vi "ObserverExample.vi"() -> ()   [LabVIEW 2025]
uses:
  ELT/Framework2.5/variantlib_code/Abstract_Actor/Abstract_Actor/Abstract_Actor.lvclass
  ELT/Framework2.5/variantlib_code/Abstract_Actor/Abstract_Actor/Abstract_Actor.lvclass/Abstract_Actor.ctl
  1c3370e3-be76-47c4-a4df-425e48d24b20.vi
  <vilib>/Utility/Data Type/NI_Data Type.lvlib
  ELT/Framework2.5/variantlib/General_Support.lvlibp
panel:
  in  "ObserverEnable":bool
  out "actorDataChanged":bool
  out "observedDataChanged":bool[](array[boolean])
  out "Cluster_out":variant[](array[variant])
  out "allActorDataName":string[](array[string])
  in  "Sender":string="pippo"
  out "Loop2":T1(array[cluster])
  out "Loop1":T1(array[cluster])
  in  "stop":bool
  out "LiveDataNames":string[](array[string])
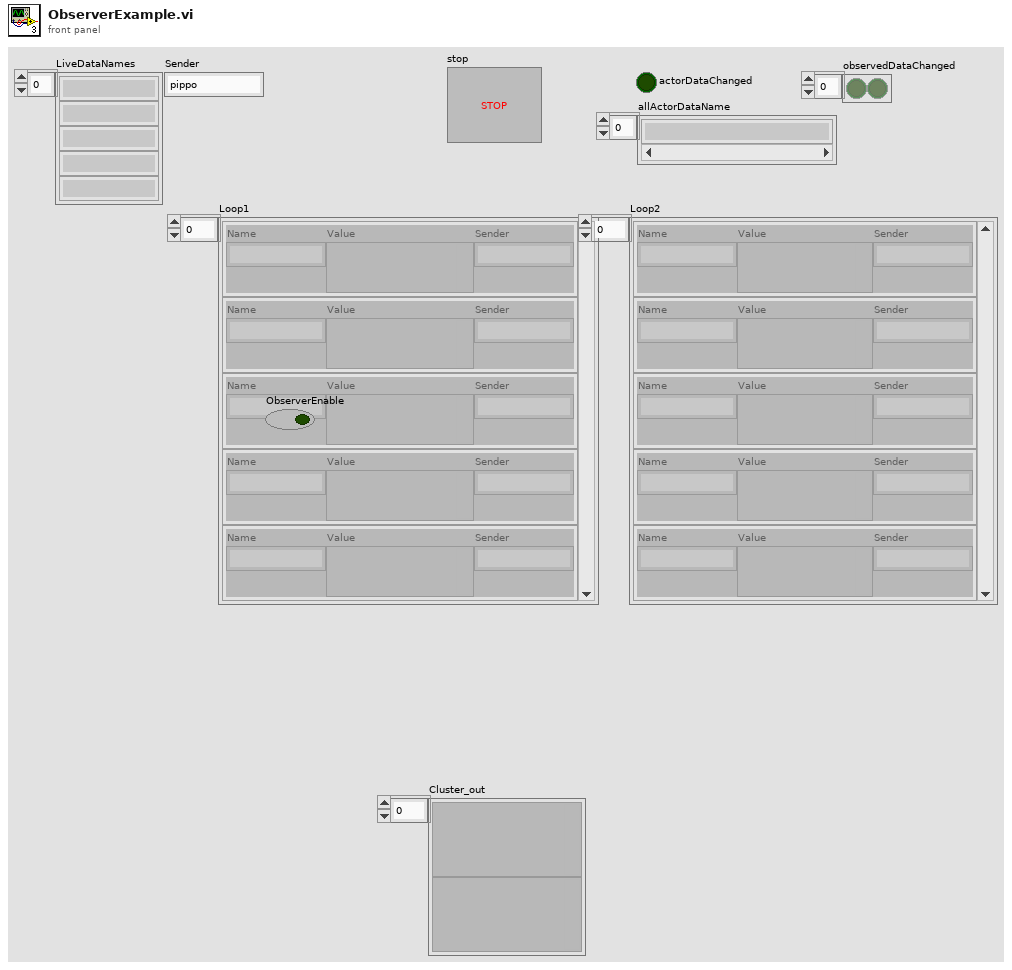
[diagram p1: front panel]
types:
  T1 = cluster{"Name":string, "Value":variant, "Sender":string}[]
  T2 = cluster{"Caller_Alias":string, "Actor_Alias":string}
  T3 = cluster{"Name":string, "Value":variant, "Sender":string}
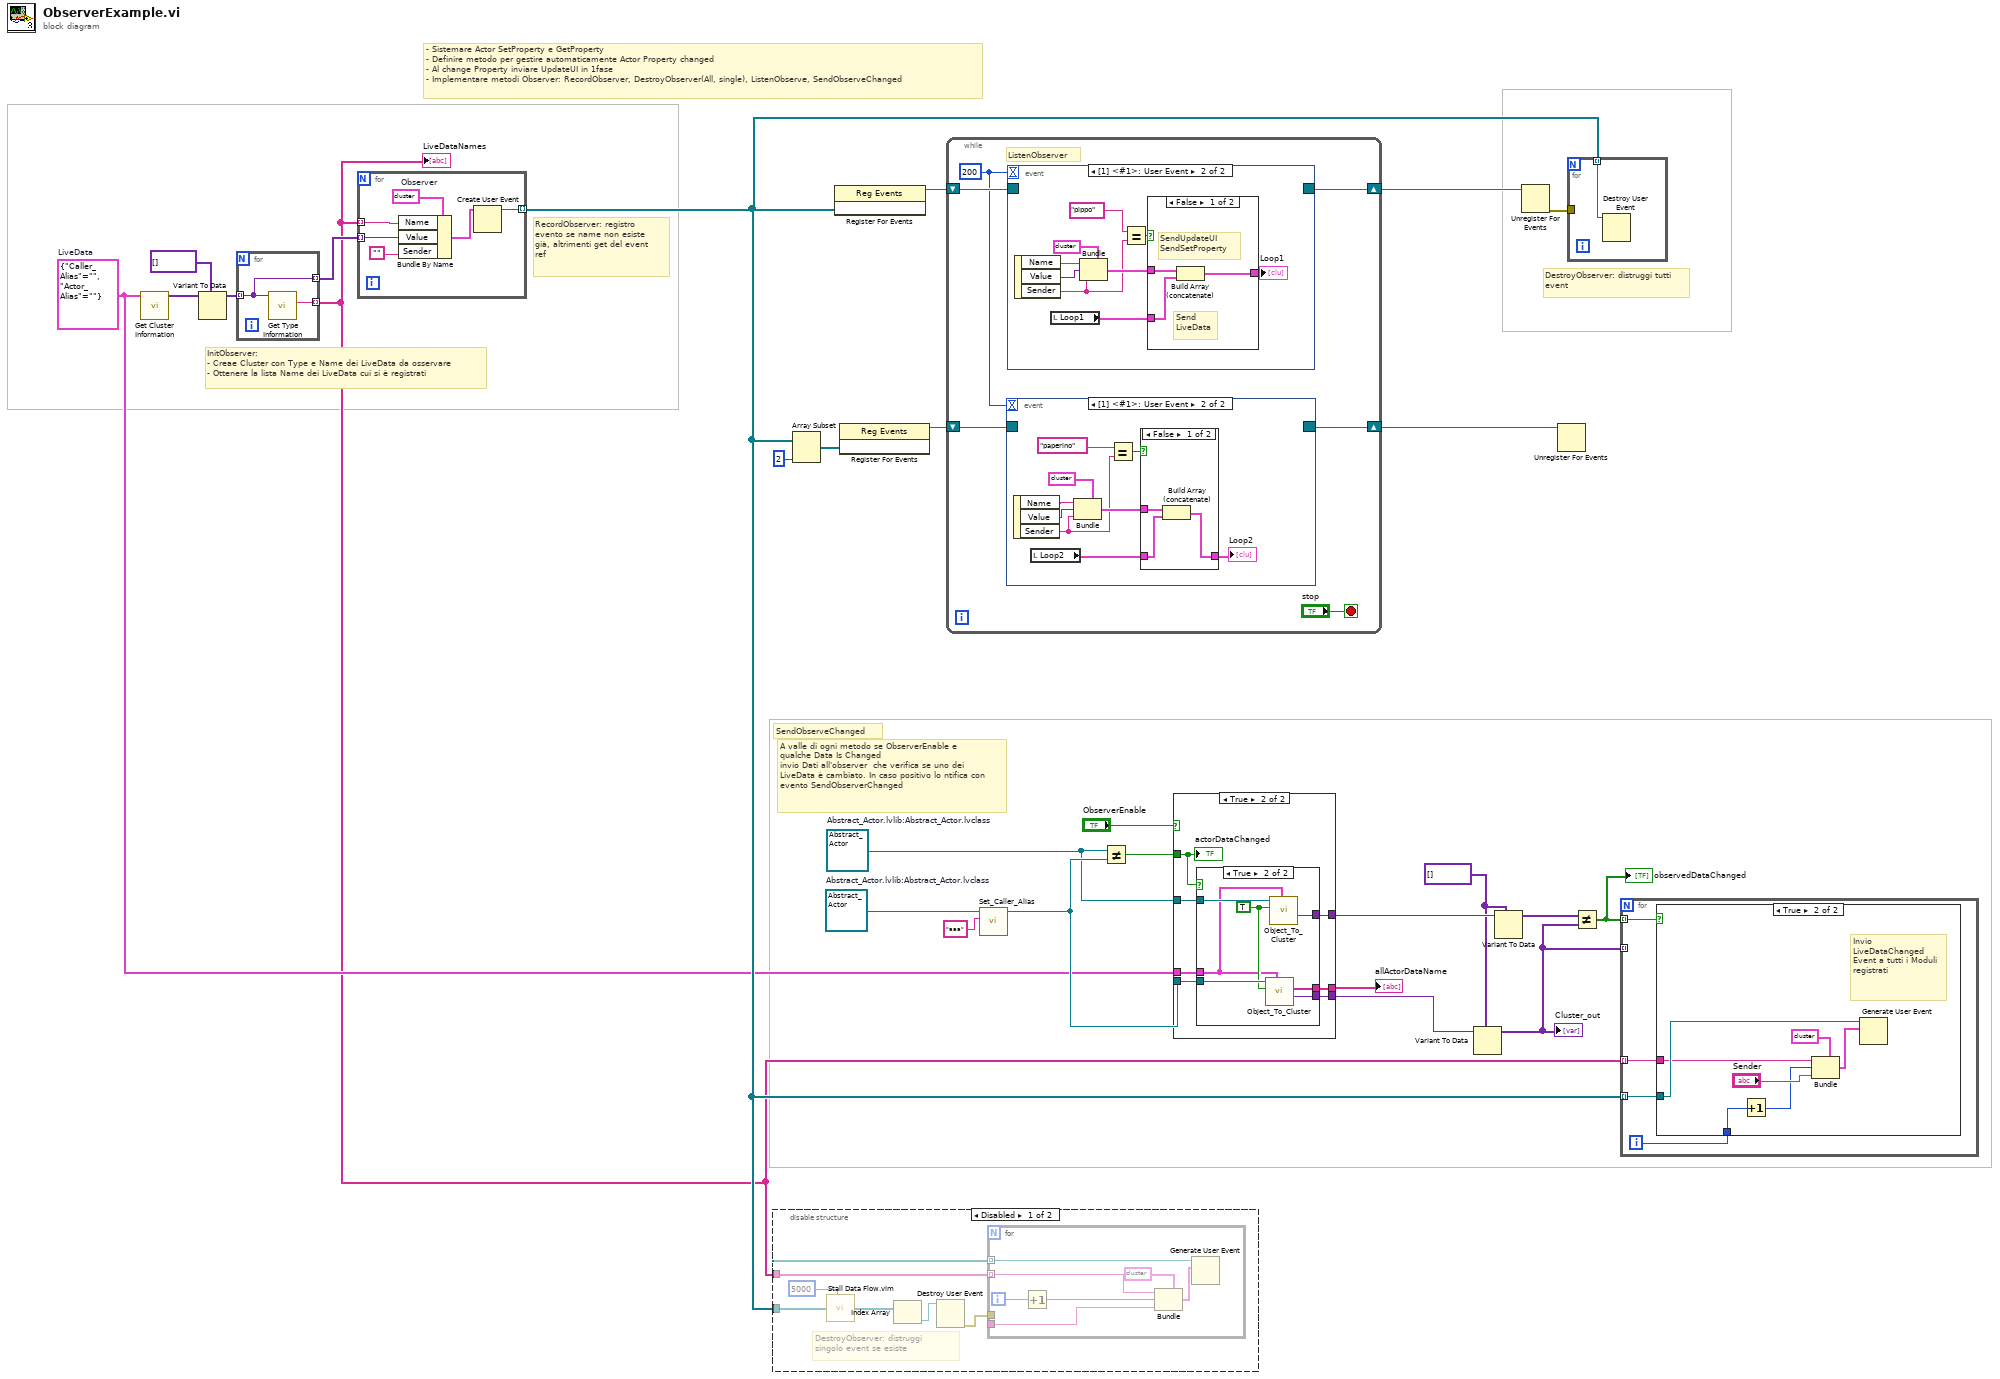
[diagram p0: block diagram]
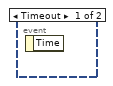
[diagram p5: hidden frame]
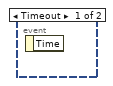
[diagram p7: hidden frame]
diagram:
  w8 = variant[] [] ("type")
  w15 = refnum<class "Abstract_Actor.lvclass"> refnum  # Abstract_Actor.lvlib:Abstract_Actor.lvclass
  w7 = refnum<class "Abstract_Actor.lvclass"> refnum  # Abstract_Actor.lvlib:Abstract_Actor.lvclass
  w2 = T2 {"Caller_Alias"="", "Actor_Alias"=""}  # LiveData
  # "A valle di ogni metodo se ObserverEnable e qualche Data Is Changed\ninvio Dati all'observer  che verifica se uno dei LiveData è cambiato. In caso positivo lo ntifica con evento SendObserverChanged"
  # "InitObserver:\n- Creae Cluster con Type e Name dei LiveData da osservare\n- Ottenere la lista Name dei LiveData cui si è registrati"
  # "SendObserveChanged"
  # "- Sistemare Actor SetProperty e GetProperty\n- Definire metodo per gestire automaticamente Actor Property changed\n- Al change Property inviare UpdateUI in 1fase\n- Implementare metodi Observer: RecordObserver, DestroyObserver(All, single), ListenObserve, SendObserveChanged"
  # "DestroyObserver: distruggi tutti event"
  # "RecordObserver: registro evento se name non esiste già, altrimenti get del event ref"
  n1 = call <vilib>:"Get Cluster Information.vi"("variant"=w2) -> ("cluster elements"=w20:variant[])  [unwired: 9 in, 1 out]
  n2 = Variant To Data(type=variant[] [], Variant=w20) -> (data=w18:variant[])  [unwired: 1 in, 1 out]
  n3 = for {
    tunnel: w18 -> [w28] mode=indexing
    tunnel: [w29] -> w1 mode=indexing
    tunnel: [w28] -> w17 mode=indexing
    n4 = call <vilib>:"Get Type Information.vi"("variant"=w28) -> ("name"=w29:string)  [unwired: 6 in, 4 out]
  }
  "LiveDataNames" <- w1
  n5 = for {
    tunnel: [w35] -> w3 mode=indexing
    tunnel: w1 -> [w33] mode=indexing
    tunnel: w17 -> [w31] mode=indexing
    w34 = T3 {"Name"="", "Value"=variant, "Sender"=""}  # Observer
    n6 = Bundle By Name(cluster=w34, "Name"=w33, "Value"=w31, "Sender"="") -> (w32:T3)
    n7 = Create User Event(user event datatype=w32) -> (user event=w35:refnum<user-event>)  [unwired: 1 in, 1 out]
  }
  n8 = disable-structure shown="Disabled" {
    disable-tunnel: w3 -> [w37 _]
    disable-tunnel: w1 -> [w36 _]
    frame Disabled {
      # "DestroyObserver: distruggi singolo event se esiste"
      n9 = call "Stall Data Flow.vim"("value in"=w37, "milliseconds to wait"=u32 5000) -> ("value out"=w40:refnum<user-event>[])  [unwired: 1 out]
      n10 = Index Array(array=w40) -> (element=w41:refnum<user-event>)  [unwired: 1 in]
      n11 = Destroy User Event(user event=w41) -> (error out=w38:errorcluster)  [unwired: 1 in]
      n12 = for {
        tunnel: w37 -> [w48] mode=indexing
        tunnel: w36 -> [w46] mode=indexing
        tunnel: w38 -> [_]
        tunnel: _ -> [w43]
        i -> [w47]
        n13 = Increment(x=w47) -> (x+1=w44:i32)
        n14 = Bundle(cluster=T3 {"Name"="", "Value"=variant, "Sender"=""} ("Observer"), "Name"=w46, "Value"=w44, "Sender"=w43) -> (w45:T3)
        n15 = Generate User Event(user event=w48, event data cluster=w45) -> ()  [unwired: 2 in, 2 out]
      }
    }
    frame Enabled {
    }
  }
  n16 = Array Subset(array=w3, length=2) -> (w22:refnum<user-event>[])  [unwired: 1 in]
  n17 = register-events(w3) -> (reference out=w25:refnum<event-registration>)  [unwired: 2 in, 1 out]
  n18 = register-events(w22) -> (reference out=w23:refnum<event-registration>)  [unwired: 2 in, 1 out]
  n19 = while {
    shift-right: [w54] -> w27
    shift-left: w25 -> [w53]
    shift-right: [w52] -> w24
    shift-left: w23 -> [w49]
    stop <- "stop" stop-if-true
    w50 = 200
    # "ListenObserver"
    n20 = event shown="[1] <#1>: User Event" {
      selector: w49 -> [_ _]
      dyn-events: [_ _] -> w52
      timeout: w50 -> [_ _]
      event Timeout {
        n21 = event-data() -> ()  [unwired: 1 in, 1 out]
      }
      event User Event {
        n22 = event-data() -> ("Name"=w62:string, "Value"=w61:variant, "Sender"=w57:string)  [unwired: 1 in]
        n23 = local read "Loop2"() -> (w59:T1)
        n24 = Bundle(cluster=T3 {"Name"="", "Value"=variant, "Sender"=""} ("Observer"), "Name"=w62, "Value"=w61, "Sender"=w57) -> (w63:T3)
        n25 = Equal?(x="paperino", y=w57) -> (x = y?=w56:bool)
        n26 = case shown="False" w56 {
          tunnel: w63 -> [w66 _]
          tunnel: [w65 w67] -> w60
          tunnel: w59 -> [w64 w67]
          frame False {
            n27 = Build Array (concatenate)(w66, w64) -> (w65:T1)
          }
          frame True {
          }
        }
        "Loop2" <- w60
      }
    }
    n28 = event shown="[1] <#1>: User Event" {
      selector: w53 -> [_ _]
      dyn-events: [_ _] -> w54
      timeout: w50 -> [_ _]
      event Timeout {
        n29 = event-data() -> ()  [unwired: 1 in, 1 out]
      }
      event User Event {
        n30 = event-data() -> ("Name"=w75:string, "Value"=w74:variant, "Sender"=w71:string)  [unwired: 1 in]
        n31 = local read "Loop1"() -> (w76:T1)
        n32 = Bundle(cluster=T3 {"Name"="", "Value"=variant, "Sender"=""} ("Observer"), "Name"=w75, "Value"=w74, "Sender"=w71) -> (w73:T3)
        n33 = Equal?(x="pippo", y=w71) -> (x = y?=w69:bool)
        n34 = case shown="False" w69 {
          tunnel: w76 -> [w79 w80]
          tunnel: w73 -> [w78 _]
          tunnel: [w77 w80] -> w72
          frame False {
            # "Send\nLiveData"
            # "SendUpdateUI\nSendSetProperty"
            n35 = Build Array (concatenate)(w78, w79) -> (w77:T1)
          }
          frame True {
          }
        }
        "Loop1" <- w72
      }
    }
  }
  n36 = call "Set_Caller_Alias.vi"("Caller_Alias"="aaa", "Abstract_Actor in"=w15) -> ("Abstract_Actor out"=w13:refnum<class "Abstract_Actor.lvclass">)  [unwired: 8 in, 1 out]
  n37 = Not Equal?(x=w7, y=w13) -> (x != y?=w16:bool)
  n38 = case shown="True" "ObserverEnable" {
    tunnel: w16 -> [_ w81]
    tunnel: w13 -> [_ w87]
    tunnel: [_ w86] -> w12
    tunnel: [_ w85] -> w11
    tunnel: [_ w84] -> w9
    tunnel: w7 -> [_ w83]
    tunnel: w2 -> [_ w82]
    frame False {
    }
    frame True {
      n39 = case shown="True" w81 {
        tunnel: w87 -> [_ w94]
        tunnel: [_ w93] -> w86
        tunnel: [_ w92] -> w85
        tunnel: [_ w91] -> w84
        tunnel: w83 -> [_ w89]
        tunnel: w82 -> [_ w88]
        frame False {
        }
        frame True {
          w90 = TRUE ("All_Hierarchy (F)")
          n40 = call "Object_To_Cluster.vi"("Cluster_Type"=w88, "All_Hierarchy (F)"=w90, "LabVIEW_Object"=w94) -> ("Cluster_out"=w91:variant, "Element_Name"=w93:string[])  [unwired: 5 in, 2 out]
          n41 = call "Object_To_Cluster.vi"("Cluster_Type"=w88, "All_Hierarchy (F)"=w90, "LabVIEW_Object"=w89) -> ("Cluster_out"=w92:variant)  [unwired: 5 in, 3 out]
        }
      }
      "actorDataChanged" <- w81
    }
  }
  "allActorDataName" <- w12
  n42 = Variant To Data(type=w8, Variant=w9) -> (data=w5:variant[])  [unwired: 1 in, 1 out]
  "Cluster_out" <- w5
  n43 = Variant To Data(type=w8, Variant=w11) -> (data=w10:variant[])  [unwired: 1 in, 1 out]
  n44 = Unregister For Events(event registration refnum=w27) -> (error out=w26:errorcluster)  [unwired: 1 in]
  n45 = Unregister For Events(event registration refnum=w24) -> ()  [unwired: 1 in, 1 out]
  n46 = for {
    tunnel: w26 -> [_]
    tunnel: w3 -> [w95] mode=indexing
    n47 = Destroy User Event(user event=w95) -> ()  [unwired: 1 in, 1 out]
  }
  n48 = Not Equal?(x=w10, y=w5) -> (x != y?=w4:bool[])
  "observedDataChanged" <- w4
  n49 = for {
    tunnel: w4 -> [w99] mode=indexing
    tunnel: w5 -> [_] mode=indexing
    tunnel: w3 -> [w98] mode=indexing
    tunnel: w1 -> [w97] mode=indexing
    i -> [w96]
    n50 = case shown="True" w99 {
      tunnel: w98 -> [_ w106]
      tunnel: w97 -> [_ w104]
      tunnel: w96 -> [_ w100]
      frame False {
      }
      frame True {
        # "Invio LiveDataChanged Event a tutti i Moduli registrati"
        n51 = Increment(x=w100) -> (x+1=w101:i32)
        n52 = Bundle(cluster=T3 {"Name"="", "Value"=variant, "Sender"=""} ("Observer"), "Name"=w104, "Value"=w101, "Sender"="Sender") -> (w103:T3)
        n53 = Generate User Event(user event=w106, event data cluster=w103) -> ()  [unwired: 2 in, 2 out]
      }
    }
  }
